vi "readWritePacket.vi"(8 "error in (no error)":errorcluster, 10 "tcpRef":refnum<k5>, 11 "tcpServer in":refnum<class "TcpServer.lvclass">) -> (0 "error out":errorcluster, 2 "tcpRef":refnum<k5>, 3 "tcpServer out":refnum<class "TcpServer.lvclass">)   [LabVIEW 2018, in "TcpServer.lvclass"]
doc: "Read incomming tcp packet from Tcp Client and send tcp packet to the Tcp Client, as commands or events."
uses:
  TcpServer.lvclass
  TcpServer.lvclass/TcpServer.ctl
panel:
  out "Packet":string
  out "loop sender":i32
  out "loop receiver":i32
  out "error tcp":errorcluster
  out "Packet In":string
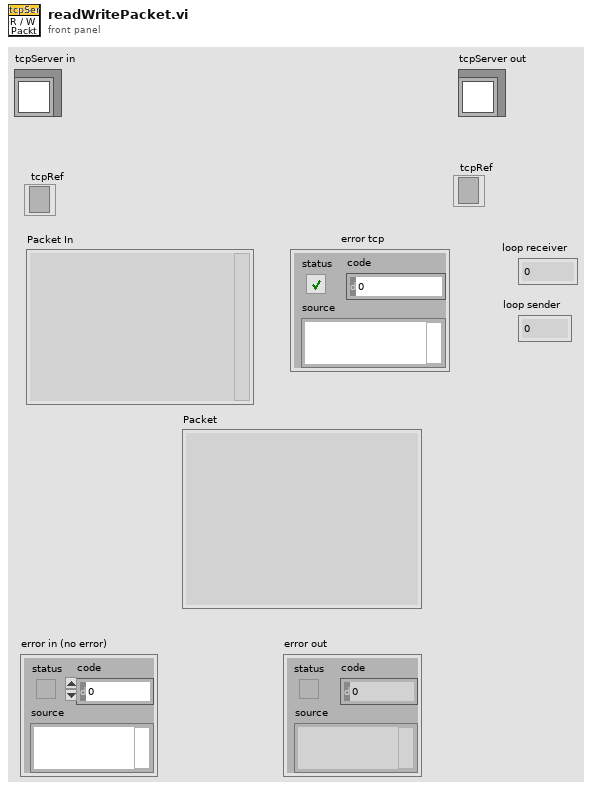
[diagram p1: front panel]
types:
  T1 = enum16{"Standard", "Buffered", "CRLF", "Immediate"}
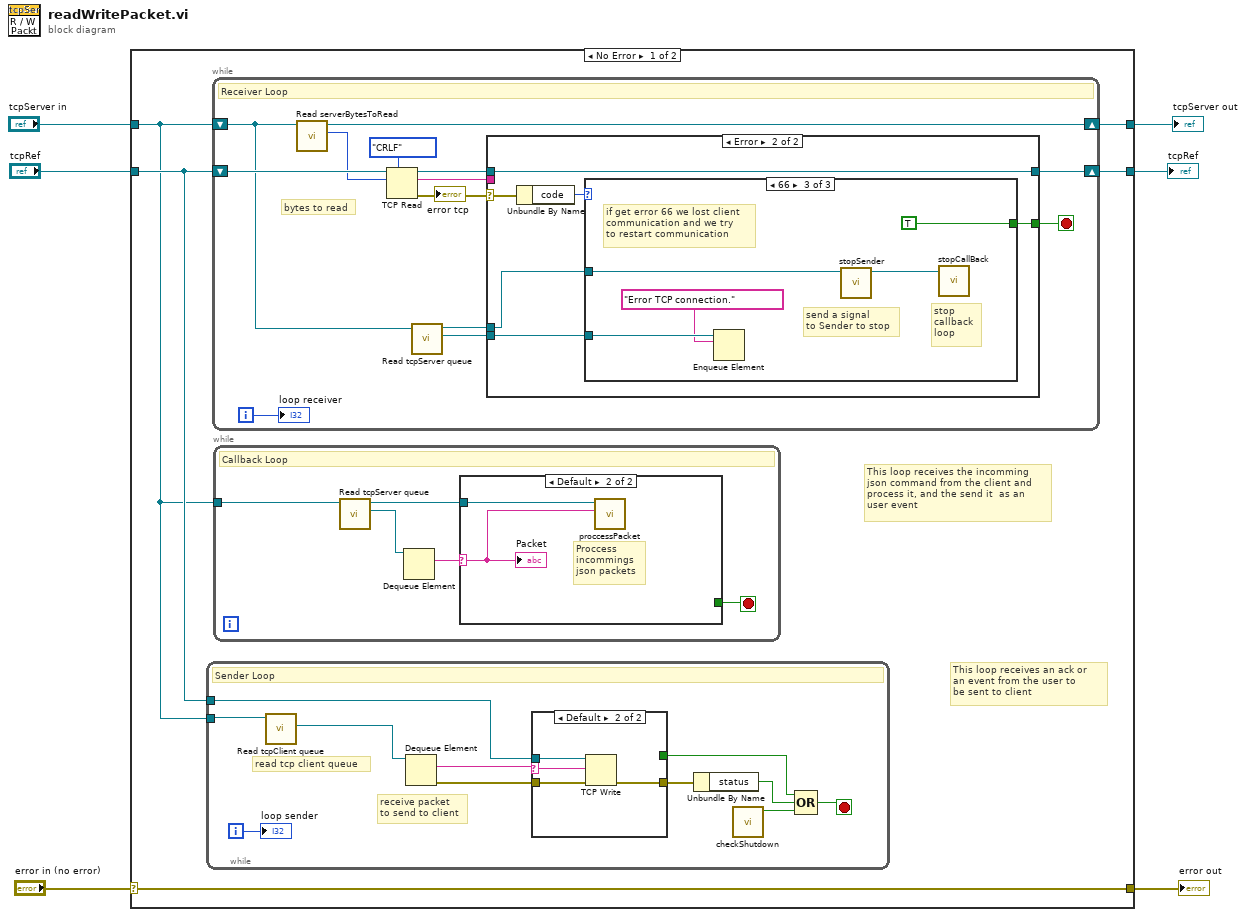
[diagram p0: block diagram]
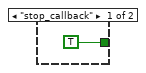
[diagram p2: hidden frame]
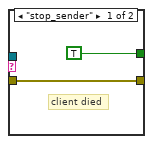
[diagram p3: hidden frame]
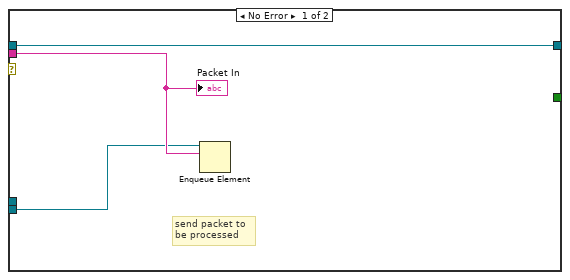
[diagram p4: hidden frame]
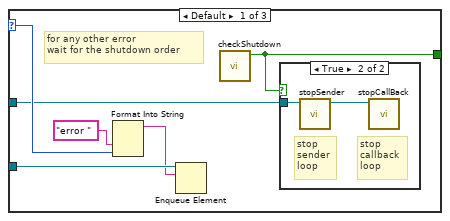
[diagram p5: hidden frame]
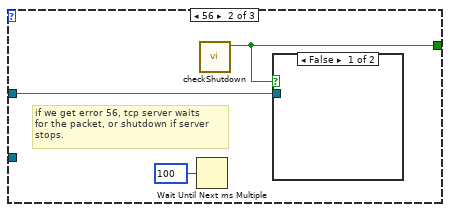
[diagram p7: hidden frame]
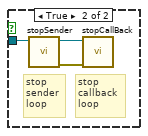
[diagram p8: hidden frame]
diagram:
  n1 = case shown="No Error" "error in (no error)" {
    selector: "error in (no error)" -> [w11 w80]
    tunnel: [w11 w80] -> w5
    tunnel: [w10 w79] -> w3
    tunnel: "tcpServer in" -> [w7 w79]
    tunnel: "tcpRef" -> [w9 w78]
    tunnel: [w8 w78] -> w1
    frame No Error {
      # "This loop receives an ack or\nan event from the user to\nbe sent to client"
      # "This loop receives the incomming\njson command from the client and\nprocess it, and the send it  as an \nuser event"
      n2 = while {
        tunnel: w7 -> [w30]
        tunnel: w9 -> [w28]
        i -> [w27]
        stop <- w22 stop-if-true
        # "receive packet\nto send to client"
        # "read tcp client queue"
        # "Sender Loop"
        n3 = call "Read tcpClient queue.vi"("tcpServer in"=w30) -> ("tcpClient queue"=w29:refnum<queue>)  [unwired: 8 in, 2 out]
        n4 = Dequeue Element(queue=w29) -> (element=w21:string, error out=w26:errorcluster)  [unwired: 2 in, 2 out]
        n5 = case shown="Default" w21 {
          selector: w21 -> [_ w33]
          tunnel: w28 -> [_ w36]
          tunnel: w26 -> [w32 w35]
          tunnel: [w32 w34] -> w25
          tunnel: [TRUE _] -> w20
          frame "stop_sender" {
            # "client died"
          }
          frame Default {
            n6 = TCP Write(connection ID=w36, data in=w33, error in (no error)=w35) -> (error out=w34:errorcluster)  [unwired: 1 in, 2 out]
          }
        }
        n7 = Unbundle By Name(w25) -> ("status"=w24:bool)
        n8 = call "checkShutdown.vi"() -> ("shutdown?"=w23:bool)  [unwired: 10 in, 1 out]
        n9 = Compound Arithmetic op=OR(w20, w24, w23) -> (w22:bool)
        "loop sender" <- w27
      }
      n10 = while {
        shift-right: [w41] -> w10
        shift-left: w7 -> [w42]
        shift-right: [w44] -> w8
        shift-left: w9 -> [w47]
        i -> [w43]
        stop <- w38 stop-if-true
        # "bytes to read"
        # "Receiver Loop"
        n11 = call "Read serverBytesToRead.vi"("tcpServer in"=w42) -> ("serverBytesToRead"=w40:i32, "tcpServer out"=w41:refnum<class "TcpServer.lvclass">)  [unwired: 8 in, 1 out]
        n12 = TCP Read(connection ID=w47, bytes to read=w40, 7:T1."CRLF" ("mode (standard)")) -> (connection ID out=w45:refnum<k5>, data out=w49:string, error out=w46:errorcluster)  [unwired: 2 in]
        "error tcp" <- w46
        n13 = call "Read tcpServer queue.vi"("tcpServer in"=w42) -> ("tcpServer queue"=w39:refnum<queue>, "tcpServer out"=w37:refnum<class "TcpServer.lvclass">)  [unwired: 8 in, 1 out]
        n14 = case shown="Error" w46 {
          selector: w46 -> [_ w57]
          tunnel: w49 -> [w52 _]
          tunnel: w45 -> [w50 w58]
          tunnel: w39 -> [w51 w55]
          tunnel: [w50 w58] -> w44
          tunnel: [_ w54] -> w38
          tunnel: w37 -> [_ w53]
          frame No Error {
            # "send packet to\nbe processed"
            n15 = Enqueue Element(queue=w51, element=w52) -> ()  [unwired: 2 in, 3 out]
            "Packet In" <- w52
          }
          frame Error {
            n16 = Unbundle By Name(w57) -> ("code"=w56:i32)
            n17 = case shown="66" w56 {
              selector: w56 -> [w63 _ _]
              tunnel: w55 -> [w62 _ w77]
              tunnel: [w59 w68 TRUE ("shutdown?")] -> w54
              tunnel: w53 -> [w60 w67 w74]
              frame Default {
                # "for any other error\nwait for the shutdown order"
                n18 = Format Into String("error ", w63) -> (resulting string=w61:string)  [unwired: 3 in, 1 out]
                n19 = Enqueue Element(queue=w62, element=w61) -> ()  [unwired: 2 in, 3 out]
                n20 = call "checkShutdown.vi"() -> ("shutdown?"=w59:bool)  [unwired: 10 in, 1 out]
                n21 = case shown="True" w59 {
                  tunnel: w60 -> [_ w66]
                  frame False {
                  }
                  frame True {
                    # "stop\ncallback\nloop"
                    # "stop\nsender\nloop"
                    n22 = call "stopSender.vi"("TcpServer in"=w66) -> ("TcpServer out"=w65:refnum<class "TcpServer.lvclass">)  [unwired: 9 in, 1 out]
                    n23 = call "stopCallBack.vi"("TcpServer in"=w65) -> ()  [unwired: 9 in, 2 out]
                  }
                }
              }
              frame 56 {
                # "if we get error 56, tcp server waits\nfor the packet, or shutdown if server\nstops."
                n24 = Wait Until Next ms Multiple(millisecond multiple=u32 100) -> ()  [unwired: 1 out]
                n25 = call "checkShutdown.vi"() -> ("shutdown?"=w68:bool)  [unwired: 10 in, 1 out]
                n26 = case shown="False" w68 {
                  tunnel: w67 -> [_ w72]
                  frame False {
                  }
                  frame True {
                    # "stop\ncallback\nloop"
                    # "stop\nsender\nloop"
                    n27 = call "stopSender.vi"("TcpServer in"=w72) -> ("error out"=w71:errorcluster, "TcpServer out"=w70:refnum<class "TcpServer.lvclass">)  [unwired: 9 in]
                    n28 = call "stopCallBack.vi"("error in (no error)"=w71, "TcpServer in"=w70) -> ()  [unwired: 8 in, 2 out]
                  }
                }
              }
              frame 66 {
                # "stop\ncallback\nloop"
                # "send a signal \nto Sender to stop"
                # "if get error 66 we lost client \ncommunication and we try\nto restart communication"
                n29 = Enqueue Element(queue=w77, element="Error TCP connection.") -> ()  [unwired: 2 in, 3 out]
                n30 = call "stopSender.vi"("TcpServer in"=w74) -> ("TcpServer out"=w73:refnum<class "TcpServer.lvclass">)  [unwired: 9 in, 1 out]
                n31 = call "stopCallBack.vi"("TcpServer in"=w73) -> ()  [unwired: 9 in, 2 out]
              }
            }
          }
        }
        "loop receiver" <- w43
      }
      n32 = while {
        tunnel: w7 -> [w13]
        stop <- w12 stop-if-true
        # "Callback Loop"
        n33 = call "Read tcpServer queue.vi"("tcpServer in"=w13) -> ("tcpServer queue"=w16:refnum<queue>, "tcpServer out"=w15:refnum<class "TcpServer.lvclass">)  [unwired: 8 in, 1 out]
        n34 = Dequeue Element(queue=w16) -> (element=w14:string)  [unwired: 2 in, 3 out]
        n35 = case shown="Default" w14 {
          selector: w14 -> [_ w18]
          tunnel: w15 -> [_ w19]
          tunnel: [TRUE _] -> w12
          frame "stop_callback" {
          }
          frame Default {
            # "Proccess\nincommings\njson packets"
            n36 = call "proccessPacket.vi"("tcp packet"=w18, "tcpServer in"=w19) -> ()  [unwired: 8 in, 2 out]
            "Packet" <- w18
          }
        }
      }
    }
    frame Error {
    }
  }
  "error out" <- w5
  "tcpServer out" <- w3
  "tcpRef" <- w1
